vi "unflattenVelocityFromXML_Array.vi"(8 "error in (no error)":errorcluster, 9 "velocityUnitInXML":T1, 10 "xmlString":string, 11 "velocityForType":dbl[unit][](array[numeric])=[0.13468124061222908, 0.26936248122445816, 0.40404372183668724, 0.5387249624489163]) -> (0 "error out":errorcluster, 3 "velocity":dbl[unit][](array[numeric]))   [LabVIEW 2012, in "UnitsAndXML.lvlib"]
uses:
  <userlib>/Common/UnitsAndXML/UnitsAndXML.lvlib
  <userlib>/Common/UnitsAndXML/FlattenItemWithUnitToXML/FlattenVelocityToXML/VelocityUnit.ctl
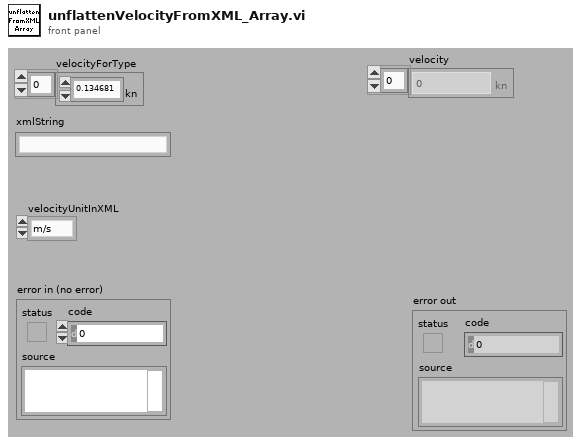
[diagram p1: front panel]
types:
  T1 = typedef "UnitsAndXML.lvlib/VelocityUnit.ctl" = enum16{"m/s", "km/s", "kn"}
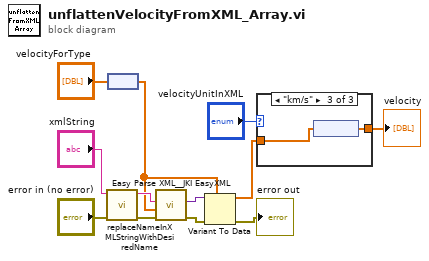
[diagram p0: block diagram]
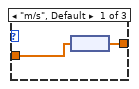
[diagram p2: hidden frame]
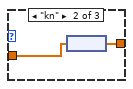
[diagram p3: hidden frame]
diagram:
  n1 = call <userlib>:"replaceNameInXMLStringWithDesiredName.vi"("error in"="error in (no error)", "xmlString"="xmlString") -> ("error out"=w1:errorcluster, "revisedXMLString"=w9:string)  [unwired: 8 in]
  n2 = node("velocityForType") -> (w8:dbl[])
  n3 = call <vilib>:"Easy Parse XML__JKI EasyXML.vi"("error in (no error)"=w1, "LabVIEW Data (Type)"=w8, "XML String"=w9) -> ("error out"=w4:errorcluster, "LabVIEW Data"=w11:variant)  [unwired: 7 in]
  n4 = Variant To Data(error in=w4, type=w8, Variant=w11) -> (data=w7:dbl[], error out=→"error out":errorcluster)
  n5 = case shown="\"km/s\"" "velocityUnitInXML" {
    tunnel: w7 -> [w13 w16 w18]
    tunnel: [w14 w15 w17] -> w6
    frame "m/s", Default {
      n6 = node(w13) -> (w14:dbl[unit][])
    }
    frame "kn" {
      n7 = node(w16) -> (w15:dbl[unit][])
    }
    frame "km/s" {
      n8 = node(w18) -> (w17:dbl[unit][])
    }
  }
  "velocity" <- w6
